vi "Save System Definition.vi"(8 "error in (no error)":errorcluster, 11 ".NET Refnum in":refnum<k24>) -> (0 "error out":errorcluster, 3 ".NET Refnum out":refnum<k24>)   [LabVIEW 2018]
uses:
  NationalInstruments.VeriStand.SystemDefinitionAPI
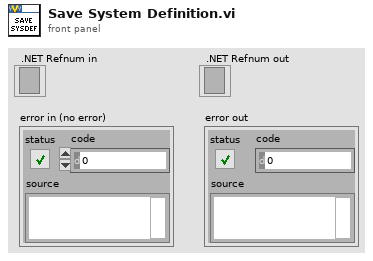
[diagram p1: front panel]
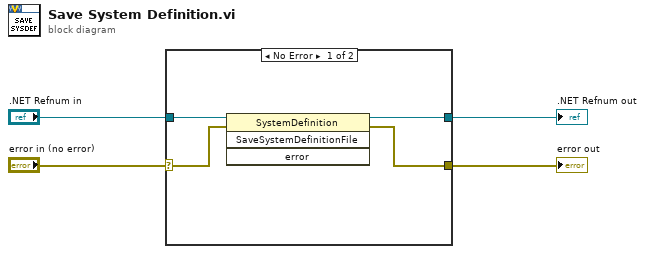
[diagram p0: block diagram]
diagram:
  n1 = case shown="No Error" "error in (no error)" {
    selector: "error in (no error)" -> [w5 w9]
    tunnel: [w8 w10] -> w4
    tunnel: [w7 w9] -> w3
    tunnel: ".NET Refnum in" -> [w6 w10]
    frame No Error {
      n2 = invoke class="SystemDefinition" method="SaveSystemDefinitionFile"(reference=w6, error in=w5) -> (reference out=w8:refnum<k24>, error out=w7:errorcluster)  [unwired: 2 in, 2 out]
    }
    frame Error {
    }
  }
  ".NET Refnum out" <- w4
  "error out" <- w3
